vi "Initialize.vi"(8 "error in (no error)":errorcluster, 11 "Stack in":refnum<class "Stack.lvclass">) -> (0 "error out":errorcluster, 3 "Stack out":refnum<class "Stack.lvclass">)   [LabVIEW 2020, in "Map Model.lvlib" / "Stack.lvclass"]
uses:
  Stack.lvclass
  Tools/Undoable Tool/Undoable Tool.lvclass
  Stack.lvclass/Stack.ctl
panel:
  # "NOTICE -- YOU MUST LEAVE THIS NOTICE IN PLACE.\n\nCopyright (c) 2017, LIANG LIU Shawn.Liu.cn@gmail.com\nAll rights reserved.\n\nRedistribution and use in source and binary forms, with or without modification, are permitted provided that the following conditions are met:\n-Redistributions of source code must retain the above copyright notice, this list of conditions and the following disclaimer.\n-Redistributions in binary form must reproduce the above copyright notice, this list of conditions and the following disclaimer in the documentation and/or other materials provided with the distribution.\n-Neither the name of the eLp nor the names of its contributors may be used to endorse or promote products derived from this software without specific prior written permission.\n\nTHIS SOFTWARE IS PROVIDED BY THE COPYRIGHT HOLDERS AND CONTRIBUTORS \"AS IS\" AND ANY EXPRESS OR IMPLIED WARRANTIES, INCLUDING, BUT NOT LIMITED TO, THE IMPLIED WARRANTIES OF MERCHANTABILITY AND FITNESS FOR A PARTICULAR PURPOSE ARE DISCLAIMED. IN NO EVENT SHALL THE COPYRIGHT HOLDER OR CONTRIBUTORS BE LIABLE FOR ANY DIRECT, INDIRECT, INCIDENTAL, SPECIAL, EXEMPLARY, OR CONSEQUENTIAL DAMAGES (INCLUDING, BUT NOT LIMITED TO, PROCUREMENT OF SUBSTITUTE GOODS OR SERVICES; LOSS OF USE, DATA, OR PROFITS; OR BUSINESS INTERRUPTION) HOWEVER CAUSED AND ON ANY THEORY OF LIABILITY, WHETHER IN CONTRACT, STRICT LIABILITY, OR TORT (INCLUDING NEGLIGENCE OR OTHERWISE) ARISING IN ANY WAY OUT OF THE USE OF THIS SOFTWARE, EVEN IF ADVISED OF THE POSSIBILITY OF SUCH DAMAGE."
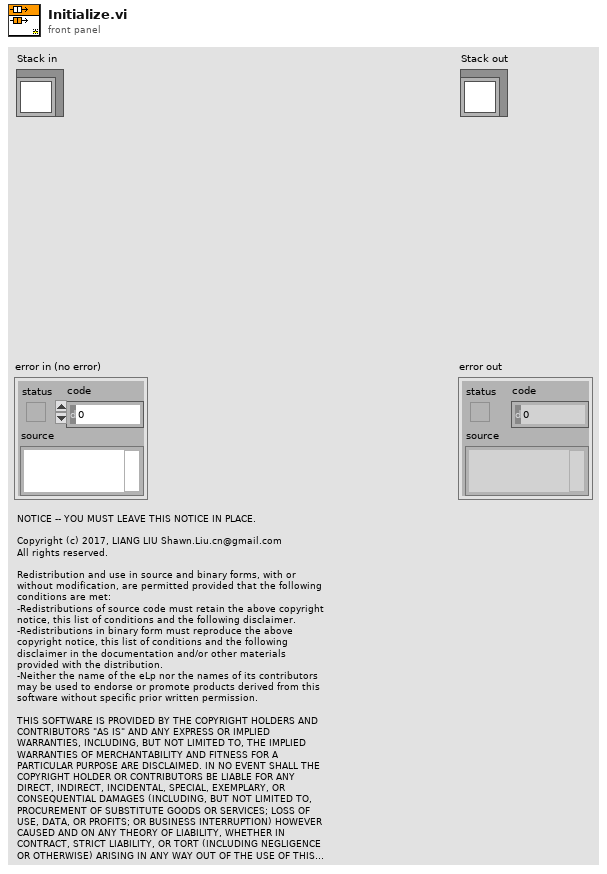
[diagram p1: front panel]
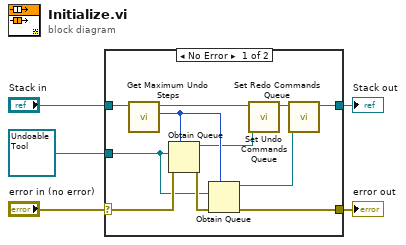
[diagram p0: block diagram]
diagram:
  n1 = case shown="No Error" "error in (no error)" {
    selector: "error in (no error)" -> [w12 w18]
    tunnel: "Stack in" -> [w16 w17]
    tunnel: refnum<class "Undoable Tool.lvclass"> refnum ("Map Model.lvlib:Undoable Tool.lvclass") -> [w6 _]
    tunnel: [w11 w18] -> w2
    tunnel: [w8 w17] -> w1
    frame No Error {
      n2 = call "Get Maximum Undo Steps.vi"("Stack in"=w16) -> ("Maximum Undo Steps"=w14:i32, "Stack out"=w15:refnum<class "Stack.lvclass">)  [unwired: 9 in]
      n3 = Obtain Queue(max queue size (-1, unlimited)=w14, element data type=w6, error in (no error)=w12) -> (queue out=w9:refnum<queue>, error out=w13:errorcluster)  [unwired: 2 in, 1 out]
      n4 = Obtain Queue(max queue size (-1, unlimited)=w14, element data type=w6, error in (no error)=w13) -> (queue out=w7:refnum<queue>, error out=w11:errorcluster)  [unwired: 2 in, 1 out]
      n5 = call "Set Undo Commands Queue.vi"("Undo Commands Queue"=w9, "Stack in"=w15) -> ("Stack out"=w10:refnum<class "Stack.lvclass">)  [unwired: 9 in]
      n6 = call "Set Redo Commands Queue.vi"("Redo Commands Queue"=w7, "Stack in"=w10) -> ("Stack out"=w8:refnum<class "Stack.lvclass">)  [unwired: 9 in]
    }
    frame Error {
    }
  }
  "error out" <- w2
  "Stack out" <- w1
